vi "MoveDistance.vi"() -> ()   [LabVIEW 2014]
uses:
  <vilib>/Rock Robotics/WPI/CAN/TalonSRX/WPI_CANTalonSRX_GlobalStatus.ctl
  <vilib>/Rock Robotics/WPI/CAN/TalonSRX/WPI_CANTalonSRX_APIControlMode.ctl
panel:
  out "Sensor Position Goto":dbl
  out "Sensor Position":dbl
  out "Talon SRX Status":T1
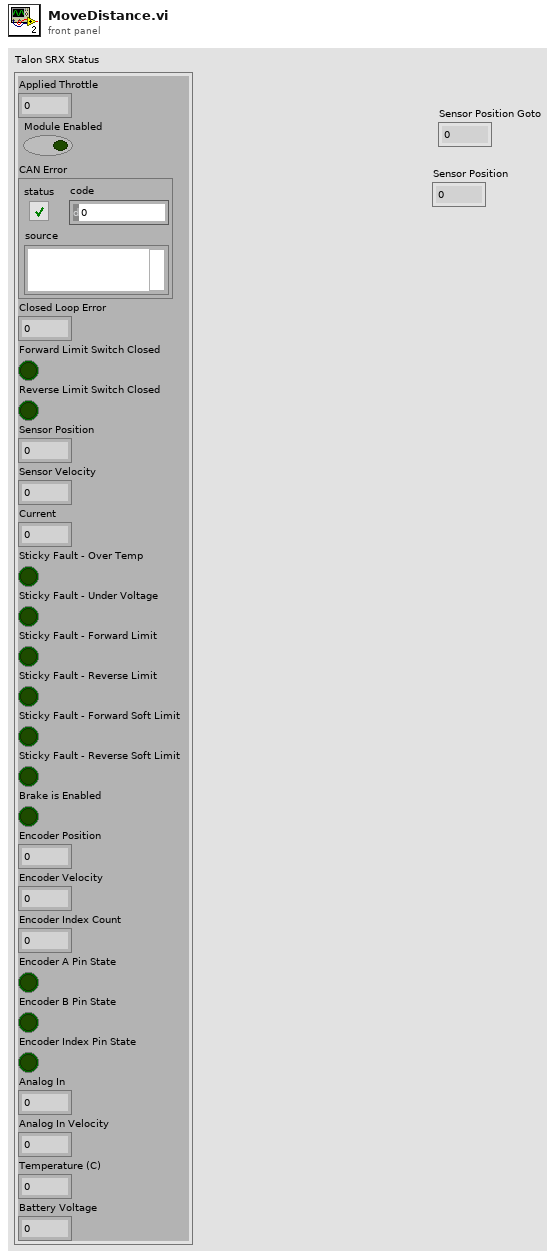
[diagram p1: front panel]
types:
  T1 = typedef "WPI_CANTalonSRX_GlobalStatus.ctl" = cluster{"Applied Throttle":dbl, "Module Enabled":bool, "CAN Error":errorcluster, "Closed Loop Error":dbl, "Forward Limit Switch Closed":bool, "Reverse Limit Switch Closed":bool, "Sensor Position":dbl, "Sensor Velocity":dbl, "Current":dbl, "Sticky Fault - Over Temp":bool, "Sticky Fault - Under Voltage":bool, "Sticky Fault - Forward Limit":bool, "Sticky Fault - Reverse Limit":bool, "Sticky Fault - Forward Soft Limit":bool, "Sticky Fault - Reverse Soft Limit":bool, "Brake is Enabled":bool, "Encoder Position":dbl, "Encoder Velocity":dbl, "Encoder Index Count":dbl, "Encoder A Pin State":bool, "Encoder B Pin State":bool, "Encoder Index Pin State":bool, "Analog In":dbl, "Analog In Velocity":dbl, "Temperature (C)":dbl, "Battery Voltage":dbl}
  T2 = typedef "WPI_CANTalonSRX_APIControlMode.ctl" = enum8{"Percent VBus", "Speed", "Position", "Slave", "Unchanged / Invalid"}
  T3 = typedef "WPI_MotorControlDeviceRef.ctl" = cluster{"DeviceStatus":errorcluster, "Type":T4, "PWM":cluster{"Controller":T5, "PWM Channel":T6, "DeadBand":T7}, "CAN":cluster{"Device Number":u8, "Control Mode":T8, "Semaphore":T9, "Max Vout":dbl, "TalonSRX Control Mode":T2}, "Invert":bool, "TransformRef":T10, "InvTransformRef":T10}
  T4 = typedef "WPI_MotorControlType.ctl" = enum16{"PWM", "CAN", "CANTalonSRX"}
  T5 = typedef "FPGA_TypedefDigitalModule.ctl" = enum16{"Controller 1"}
  T6 = typedef "FPGA_DIOPWMChannel.ctl" = enum8{"PWM 0", "PWM 1", "PWM 2", "PWM 3", "PWM 4", "PWM 5", "PWM 6", "PWM 7", "PWM 8", "PWM 9", "PWM MXP 0", "PWM MXP 1", "PWM MXP 2", "PWM MXP 3", "PWM MXP 4", "PWM MXP 5", "PWM MXP 6", "PWM MXP 7", "PWM MXP 8", "PWM MXP 9", "Invalid"}
  T7 = typedef "WPI_PWMDeadband.ctl" = cluster{"Name":string, "maxPositivePwm":i32, "minPositivePwm":i32, "centerPwm":i32, "maxNegativePwm":i32, "minNegativePwm":i32, "angularRange":u16}
  T8 = typedef "WPI_CANJaguar_ControlMode.ctl" = enum8{"Percent VBus", "Current", "Speed", "Position", "Voltage"}
  T9 = typedef "Semaphore RefNum" = refnum<k1>
  T10 = typedef "WPI_PWMTransform_ConPane.ctl" = refnum<vi>
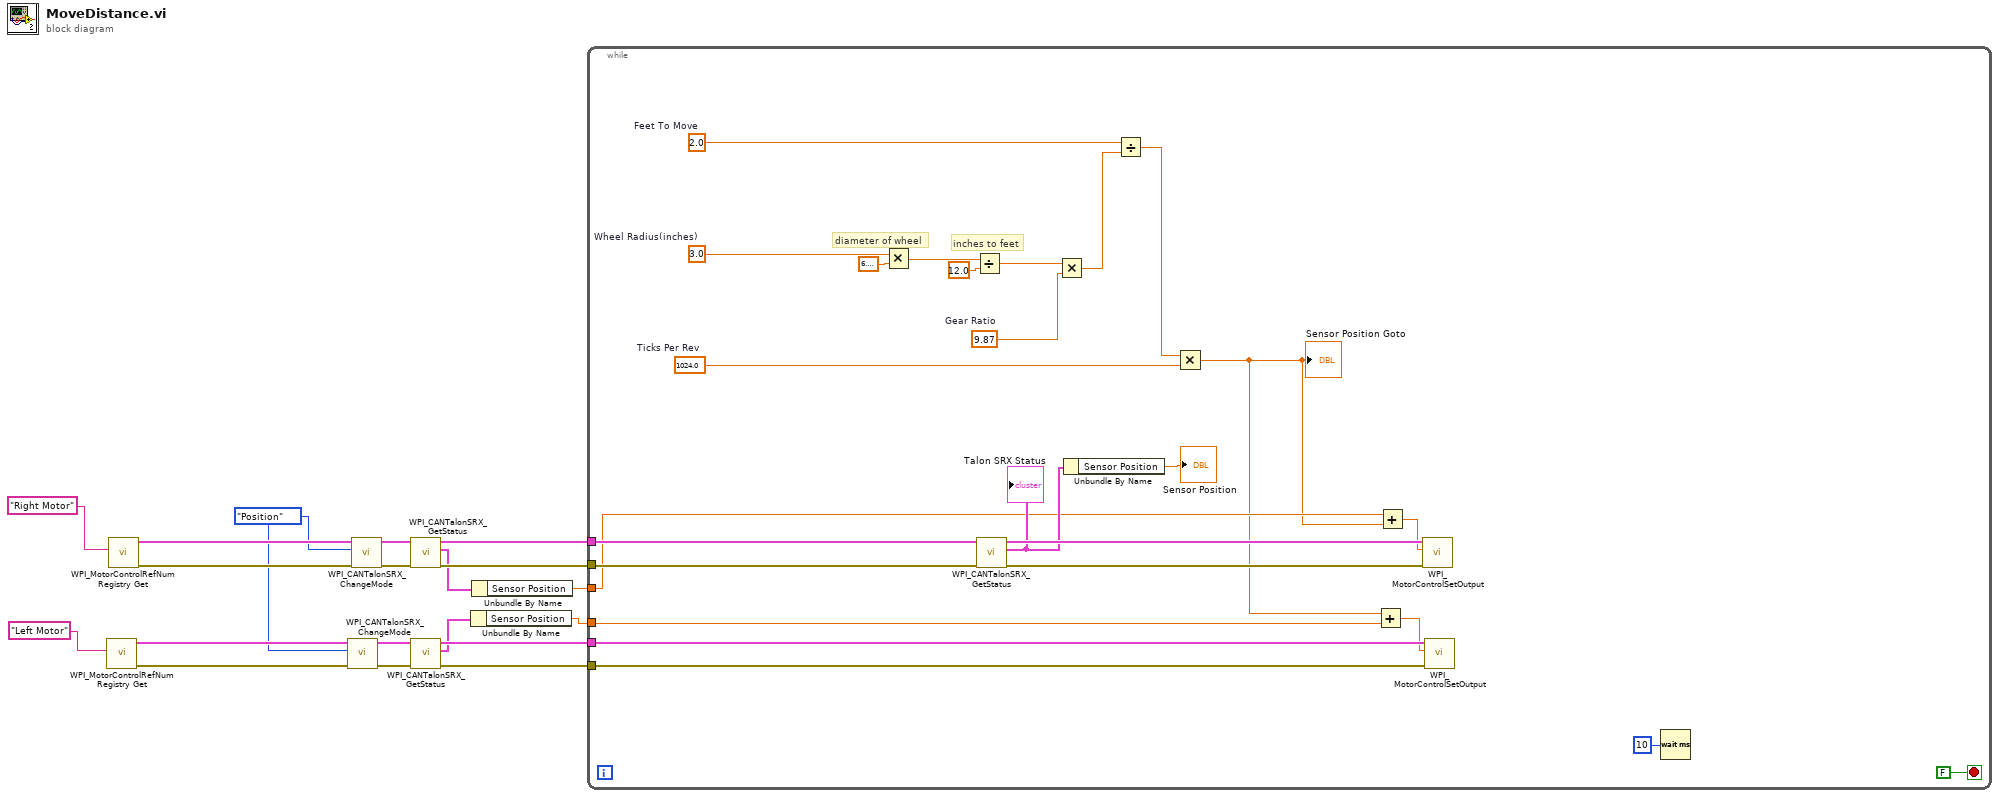
[diagram p0: block diagram]
diagram:
  w13 = WPI_CANTalonSRX_APIControlMode."Position" ("Control Mode")
  n1 = call <vilib>:"WPI_MotorControlRefNum Registry Get.vi"("refnum name"="Left Motor") -> ("error out"=w14:errorcluster, "MotorControlDevRef"=w15:T3)  [unwired: 9 in]
  n2 = call <vilib>:"WPI_MotorControlRefNum Registry Get.vi"("refnum name"="Right Motor") -> ("error out"=w16:errorcluster, "MotorControlDevRef"=w17:T3)  [unwired: 9 in]
  n3 = call <vilib>:"WPI_CANTalonSRX_ChangeMode.vi"("error in (no error)"=w14, "Control Mode"=w13, "CAN Talon SRX Ref"=w15) -> ("error out"=w5:errorcluster, "CAN Talon SRX Ref Out"=w6:T3)  [unwired: 7 in]
  n4 = call <vilib>:"WPI_CANTalonSRX_ChangeMode.vi"("error in (no error)"=w16, "Control Mode"=w13, "CAN Talon SRX Ref"=w17) -> ("error out"=w11:errorcluster, "CAN Talon SRX Ref Out"=w12:T3)  [unwired: 7 in]
  n5 = call <vilib>:"WPI_CANTalonSRX_GetStatus.vi"("error in (no error)"=w11, "CAN Talon SRX Ref"=w12) -> ("error out"=w10:errorcluster, "Talon SRX Status"=w8:T1, "CAN Talon SRX Ref Out"=w9:T3)  [unwired: 7 in]
  n6 = call <vilib>:"WPI_CANTalonSRX_GetStatus.vi"("error in (no error)"=w5, "CAN Talon SRX Ref"=w6) -> ("error out"=w3:errorcluster, "Talon SRX Status"=w2:T1, "CAN Talon SRX Ref Out"=w4:T3)  [unwired: 7 in]
  n7 = Unbundle By Name(w2) -> ("Sensor Position"=w1:dbl)
  n8 = Unbundle By Name(w8) -> ("Sensor Position"=w7:dbl)
  n9 = while {
    tunnel: w9 -> [w29]
    tunnel: w10 -> [w28]
    tunnel: w7 -> [w26]
    tunnel: w4 -> [w24]
    tunnel: w3 -> [w23]
    tunnel: w1 -> [w21]
    stop <- FALSE stop-if-true
    w39 = 1024.0  # Ticks Per Rev
    w44 = 3.0  # Wheel Radius(inches)
    w38 = 2.0  # Feet To Move
    w37 = 9.87  # Gear Ratio
    # "diameter of wheel"
    # "inches to feet"
    n10 = Multiply(x=w44, y=6.283185307179586) -> (x*y=w42:dbl)
    n11 = Divide(x=w42, y=12.0) -> (x/y=w36:dbl)
    n12 = call <vilib>:"WPI_CANTalonSRX_GetStatus.vi"("error in (no error)"=w28, "CAN Talon SRX Ref"=w29) -> ("error out"=w33:errorcluster, "Talon SRX Status"=w31:T1, "CAN Talon SRX Ref Out"=w34:T3)  [unwired: 7 in]
    "Talon SRX Status" <- w31
    n13 = Multiply(x=w36, y=w37) -> (x*y=w35:dbl)
    n14 = Unbundle By Name(w31) -> ("Sensor Position"=→"Sensor Position":dbl)
    n15 = Divide(x=w38, y=w35) -> (x/y=w40:dbl)
    n16 = Multiply(x=w40, y=w39) -> (x*y=w20:dbl)
    "Sensor Position Goto" <- w20
    n17 = Add(x=w20, y=w21) -> (x+y=w22:dbl)
    n18 = Add(x=w26, y=w20) -> (x+y=w25:dbl)
    n19 = call <vilib>:"WPI_MotorControlSetOutput.vi"("error in (no error)"=w33, "Output"=w25, "MotorControlDevRef"=w34) -> ()  [unwired: 6 in, 3 out]
    n20 = call <vilib>:"WPI_MotorControlSetOutput.vi"("error in (no error)"=w23, "Output"=w22, "MotorControlDevRef"=w24) -> ()  [unwired: 6 in, 3 out]
    n21 = Wait (ms)(milliseconds to wait=u32 10) -> ()  [unwired: 1 out]
  }
